vi "VCS Import Parameter.vi"(0 "axis in":cluster{"keyHandle":u32, "nodeId":u16}={"keyHandle"=0, "nodeId"=1}, 5 "import":T1 {"showMsg" items=["false", "true"]; "showDlg" items=["false", "true"]}, 11 "error in (no error)":errorcluster) -> (4 "axis out":cluster{"keyHandle":u32, "nodeId":u16}={"keyHandle"=0, "nodeId"=1}, 15 "error out":errorcluster)   [LabVIEW 2018]
doc: "<B>VCS_ImportParameter</B> writes parameters from a file to the device."
uses:
  Resources/EposCmd64.dll
  Resources/EposCmd.dll
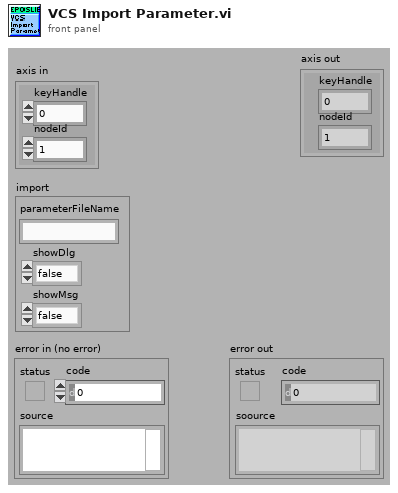
[diagram p1: front panel]
types:
  T1 = cluster{"parameterFileName":string, "showDlg":i32, "showMsg":i32}
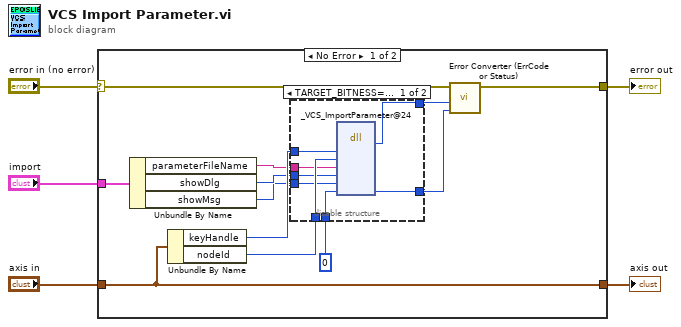
[diagram p0: block diagram]
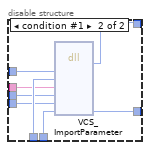
[diagram p2: hidden frame]
diagram:
  n1 = case shown="No Error" "error in (no error)" {
    selector: "error in (no error)" -> [w15 w34]
    tunnel: "axis in" -> [w17 w35]
    tunnel: [w17 w35] -> w4
    tunnel: [w16 w34] -> w3
    tunnel: "import" -> [w7 _]
    frame No Error {
      n2 = Unbundle By Name(w7) -> ("parameterFileName"=w6:string, "showDlg"=w9:i32, "showMsg"=w8:i32)
      n3 = Unbundle By Name(w17) -> ("keyHandle"=w13:u32, "nodeId"=w12:u16)
      n4 = disable-structure shown="TARGET_BITNESS==32, Standard" {
        disable-tunnel: u32 0 ("pErrorCode") -> [w25 w33]
        disable-tunnel: w13 -> [w24 w32]
        disable-tunnel: w12 -> [w23 w31]
        disable-tunnel: [w22 w30] -> w11
        disable-tunnel: [w21 w29] -> w10
        disable-tunnel: w9 -> [w20 w28]
        disable-tunnel: w8 -> [w19 w27]
        disable-tunnel: w6 -> [w18 w26]
        frame condition #0 (active) {
          n5 = dll-call lib="C:/Projeto em LabVIEW/EPOS-LabVIEW-Instrument-Driver-En/LabVIEW/maxon EPOS/Resources/EposCmd.dll" fn="_VCS_ImportParameter@24"("KeyHandle"=w24, "NodeId"=w23, "pParameterFileName"=w18, "ShowDlg"=w20, "ShowMsg"=w19, "pErrorCode"=w25) -> ("Rückgabetyp"=w22:i32, "pErrorCode"=w21:u32)  [unwired: 8 in, 2 out]
        }
        frame condition #1 {
          n6 = dll-call lib="C:/Temp/Tests/LabVIEW/maxon EPOS/Resources/EposCmd64.*" fn="VCS_ImportParameter" ("EposCmd.dll:_VCS_ImportParameter@24")("KeyHandle"=w32, "NodeId"=w31, "pParameterFileName"=w26, "ShowDlg"=w28, "ShowMsg"=w27, "pErrorCode"=w33) -> ("Rückgabetyp"=w30:i32, "pErrorCode"=w29:u32)  [unwired: 8 in, 2 out]
        }
      }
      n7 = call "Error Converter (ErrCode or Status).vi"("error code"=w10, "return type"=w11, "error in (no error)"=w15) -> ("error out"=w16:errorcluster)  [unwired: 7 in]
    }
    frame Error {
    }
  }
  "error out" <- w3
  "axis out" <- w4
